vi "peakFinding removeBaseline.vi"(8 "error in (no error)":errorcluster, 11 "sourceData":cluster{"xData":dbl[], "yData":dbl[]}) -> (0 "error out":errorcluster, 3 "signalData":cluster{"xData":dbl[], "newYData":dbl[]}, 4 "residue":dbl[](array[numeric]))   [LabVIEW 2018]
uses:
  <vilib>/Analysis/6fits.llb/Curve Fitting Criteria.ctl
  <vilib>/Analysis/NI_AALPro.lvlib
panel:
  in  "method":T1=1 items=["Least Square", "Least Absolute Residual", "Bisquare"]
  in  "polynomial order":i32=-1
  in  "iteration":i32=30
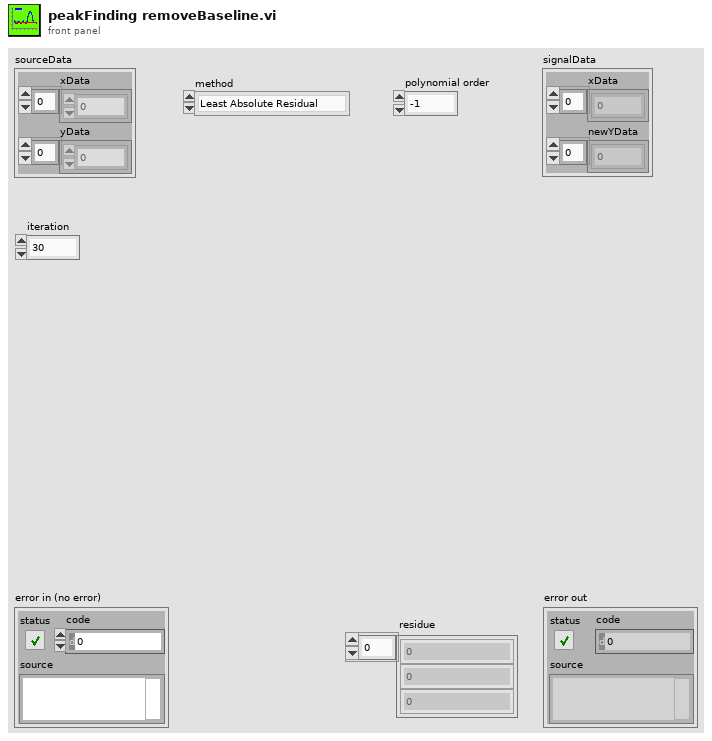
[diagram p1: front panel]
types:
  T1 = typedef "NI_AALPro.lvlib/Curve Fitting Criteria.ctl" = u16
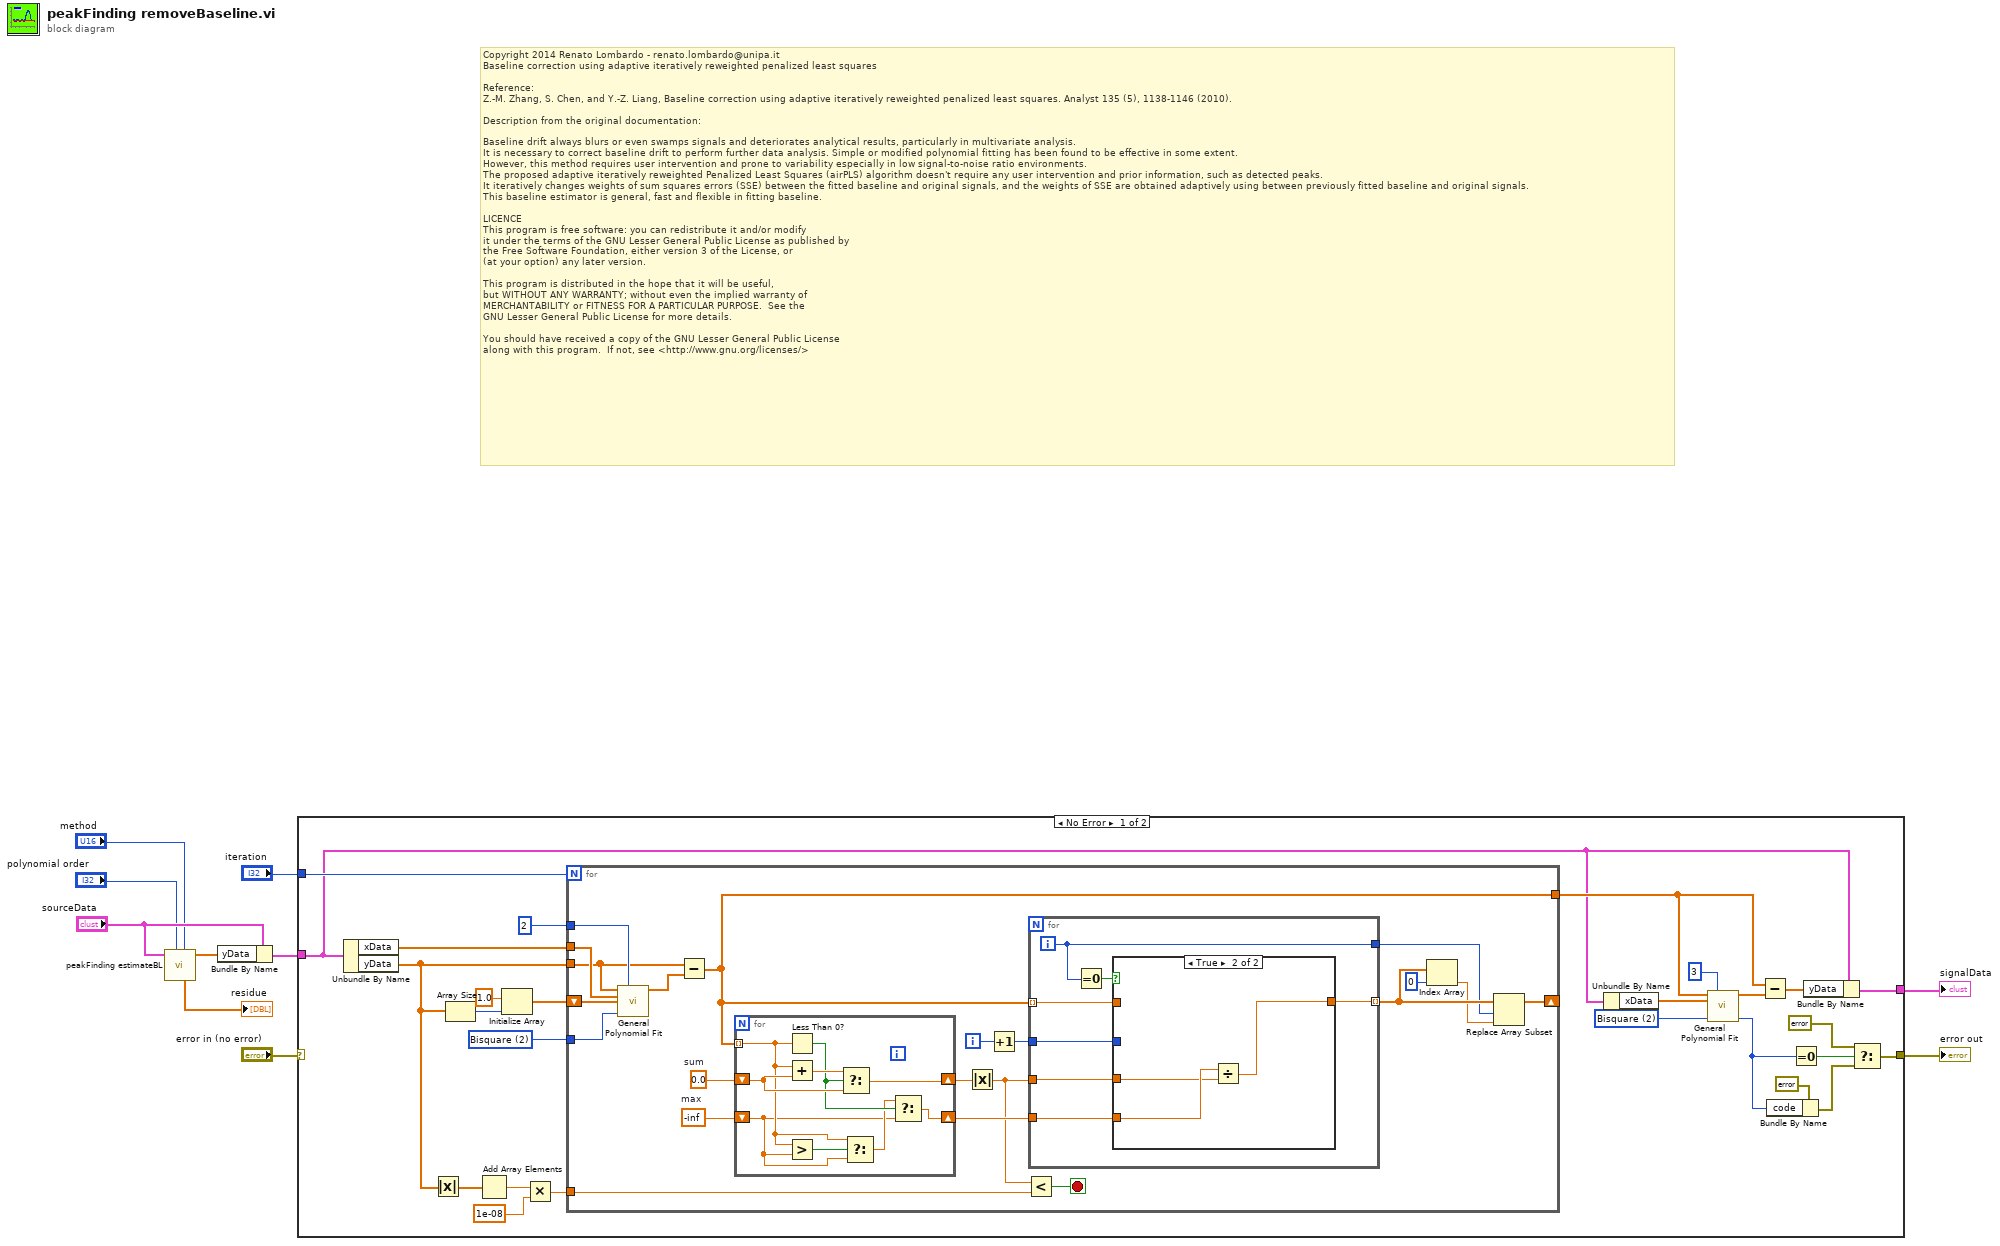
[diagram p0: block diagram]
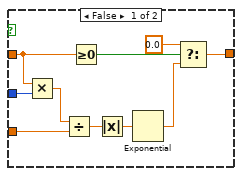
[diagram p2: hidden frame]
diagram:
  # "Copyright 2014 Renato Lombardo - renato.lombardo@unipa.it\nBaseline correction using adaptive iteratively reweighted penalized least squares\n\nReference:\nZ.-M. Zhang, S. Chen, and Y.-Z. Liang, Baseline correction using adaptive iteratively reweighted penalized least squares. Analyst 135 (5), 1138-1146 (2010).\n\nDescription from the original documentation:\n\nBaseline drift always blurs or even swamps signals and deteriorates analytical results, particularly in multivariate analysis.  \nIt is necessary to correct baseline drift to perform further data analysis. Simple or modified polynomial fitting has been found to be effective in some extent. \nHowever, this method requires user intervention and prone to variability especially in low signal-to-noise ratio environments. \nThe proposed adaptive iteratively reweighted Penalized Least Squares (airPLS) algorithm doesn't require any user intervention and prior information, such as detected peaks. \nIt iteratively changes weights of sum squares errors (SSE) between the fitted baseline and original signals, and the weights of SSE are obtained adaptively using between previously fitted baseline and original signals. \nThis baseline estimator is general, fast and flexible in fitting baseline.\n\nLICENCE\nThis program is free software: you can redistribute it and/or modify\nit under the terms of the GNU Lesser General Public License as published by\nthe Free Software Foundation, either version 3 of the License, or\n(at your option) any later version.\n\nThis program is distributed in the hope that it will be useful,\nbut WITHOUT ANY WARRANTY; without even the implied warranty of\nMERCHANTABILITY or FITNESS FOR A PARTICULAR PURPOSE.  See the\nGNU Lesser General Public License for more details.\n\nYou should have received a copy of the GNU Lesser General Public License\nalong with this program.  If not, see <http://www.gnu.org/licenses/>"
  n1 = call "peakFinding estimateBL.vi"("method"="method", "polynomial order"="polynomial order", "sourceData"="sourceData") -> ("estimateData"=w5:dbl[], "residues"=→"residue":dbl[])  [unwired: 7 in]
  n2 = Bundle By Name(cluster="sourceData", "yData"=w5) -> (w7:cluster{"xData":dbl[], "yData":dbl[]})
  n3 = case shown="No Error" "error in (no error)" {
    selector: "error in (no error)" -> [_ w87]
    tunnel: "iteration" -> [w36 _]
    tunnel: [w32 _] -> w1
    tunnel: w7 -> [w11 _]
    tunnel: [w18 w87] -> w9
    frame No Error {
      w13 = T1 2 items=["Least Square", "Least Absolute Residual", "Bisquare"] ("method")
      w17 = T1 2 items=["Least Square", "Least Absolute Residual", "Bisquare"] ("method")
      n4 = Unbundle By Name(w11) -> ("xData"=w15:dbl[], "yData"=w14:dbl[])
      n5 = Absolute Value(x=w14) -> (abs(x)=w31:dbl[])
      n6 = Array Size(array=w14) -> (size(s)=w34:i32)
      n7 = Add Array Elements(numeric array=w31) -> (sum=w30:dbl)
      n8 = Initialize Array(1.0 ("element"), w34) -> (w33:dbl[])
      n9 = Multiply(x=w30, y=1e-08) -> (x*y=w28:dbl)
      n10 = for {
        N: w36 -> [_]
        shift-right: [w41] -> _
        shift-left: w33 -> [w57]
        tunnel: w28 -> [w46]
        tunnel: [w40] -> w16
        tunnel: 2 ("polynomial order") -> [w44]
        tunnel: w15 -> [w43]
        tunnel: w14 -> [w42]
        tunnel: w13 -> [w37]
        i -> [w38]
        stop <- w45 stop-if-true
        w53 = -inf  # max
        w55 = 0.0  # sum
        n11 = call <vilib>:"General Polynomial Fit.vi"("Y"=w42, "polynomial order"=w44, "X"=w43, "Weight"=w57, "method"=w37) -> ("Best Polynomial Fit"=w56:dbl[])  [unwired: 7 in, 3 out]
        n12 = Subtract(x=w42, y=w56) -> (x-y=w40:dbl[])
        n13 = for {
          tunnel: w40 -> [w81] mode=indexing
          shift-right: [w85] -> w54
          shift-left: w55 -> [w84]
          shift-right: [w78] -> w52
          shift-left: w53 -> [w79]
          n14 = Less Than 0?(x=w81) -> (x < 0?=w83:bool)
          n15 = Add(x=w81, y=w84) -> (x+y=w86:dbl)
          n16 = Greater?(x=w81, y=w79) -> (0:w82:bool)
          n17 = Select(t=w86, s=w83, f=w84) -> (s? t:f=w85:dbl)
          n18 = Select(t=w81, s=w82, f=w79) -> (s? t:f=w80:dbl)
          n19 = Select(t=w80, s=w83, f=w79) -> (s? t:f=w78:dbl)
        }
        n20 = Absolute Value(x=w54) -> (abs(x)=w47:dbl)
        n21 = Increment(x=w38) -> (x+1=w39:i32)
        n22 = Less?(x=w47, y=w46) -> (x < y?=w45:bool)
        n23 = for {
          tunnel: w40 -> [w62] mode=indexing
          tunnel: [w64] -> w51 mode=indexing
          tunnel: w39 -> [w61]
          tunnel: w47 -> [w63]
          tunnel: [w59] -> w49
          tunnel: w52 -> [w60]
          i -> [w59]
          n24 = Equal To 0?(x=w59) -> (x = 0?=w58:bool)
          n25 = case shown="True" w58 {
            tunnel: [w72 w75] -> w64
            tunnel: w63 -> [w71 w76]
            tunnel: w62 -> [w70 _]
            tunnel: w61 -> [w69 _]
            tunnel: w60 -> [_ w77]
            frame False {
              n26 = Multiply(x=w70, y=w69) -> (x*y=w68:dbl)
              n27 = Divide(x=w68, y=w71) -> (x/y=w65:dbl)
              n28 = Greater Or Equal To 0?(x=w70) -> (x >= 0?=w74:bool)
              n29 = Absolute Value(x=w65) -> (abs(x)=w66:dbl)
              n30 = Exponential(1:w66) -> (0:w67:dbl)
              n31 = Select(t=0.0, s=w74, f=w67) -> (s? t:f=w72:dbl)
            }
            frame True {
              n32 = Divide(x=w77, y=w76) -> (x/y=w75:dbl)
            }
          }
        }
        n33 = Index Array(array=w51, index=0) -> (element=w48:dbl)
        n34 = Replace Array Subset(array=w51, new element=w48, index=w49) -> (w41:dbl[])
      }
      n35 = Unbundle By Name(w11) -> ("xData"=w24:dbl[])
      n36 = call <vilib>:"General Polynomial Fit.vi"("Y"=w16, "polynomial order"=3, "X"=w24, "method"=w17) -> ("Best Polynomial Fit"=w26:dbl[], "error"=w21:i32)  [unwired: 8 in, 2 out]
      n37 = Subtract(x=w16, y=w26) -> (x-y=w25:dbl[])
      n38 = Bundle By Name(cluster=errorcluster {"status"=TRUE, "code"=0, "source"=""} ("error in (no error)"), "code"=w21) -> (w20:errorcluster)
      n39 = Equal To 0?(x=w21) -> (x = 0?=w23:bool)
      n40 = Bundle By Name(cluster=w11, "yData"=w25) -> (w32:cluster{"xData":dbl[], "yData":dbl[]})
      n41 = Select(t=errorcluster {"status"=FALSE, "code"=0, "source"=""} ("error in (no error)"), s=w23, f=w20) -> (s? t:f=w18:errorcluster)
    }
    frame Error {
    }
  }
  "signalData" <- w1
  "error out" <- w9
